vi "CleanUp.vi"(8 "error in (no error)":errorcluster, 11 "Prueba08 in":refnum<class "Prueba031.lvclass">) -> (0 "error out":errorcluster, 3 "Prueba08 out":refnum<class "Prueba031.lvclass">)   [LabVIEW 2019, in "Prueba031.lvclass"]
uses:
  Prueba031.lvclass
  Prueba031.lvclass/Prueba031.ctl
panel:
  out "Tabla_int":string[][](array[string])
  out "Tabla_ext":string[][](array[string])
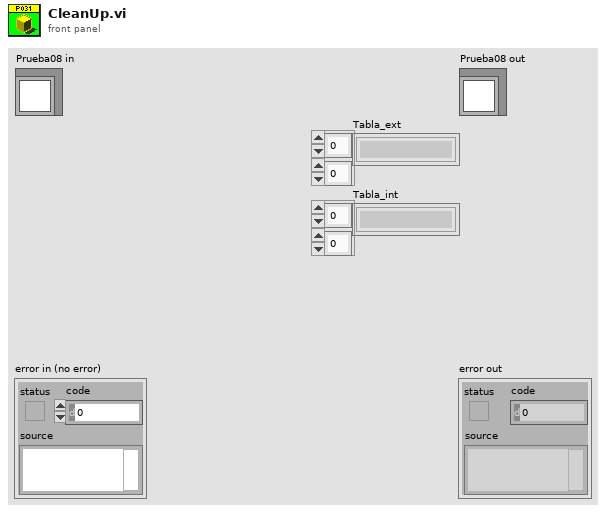
[diagram p1: front panel]
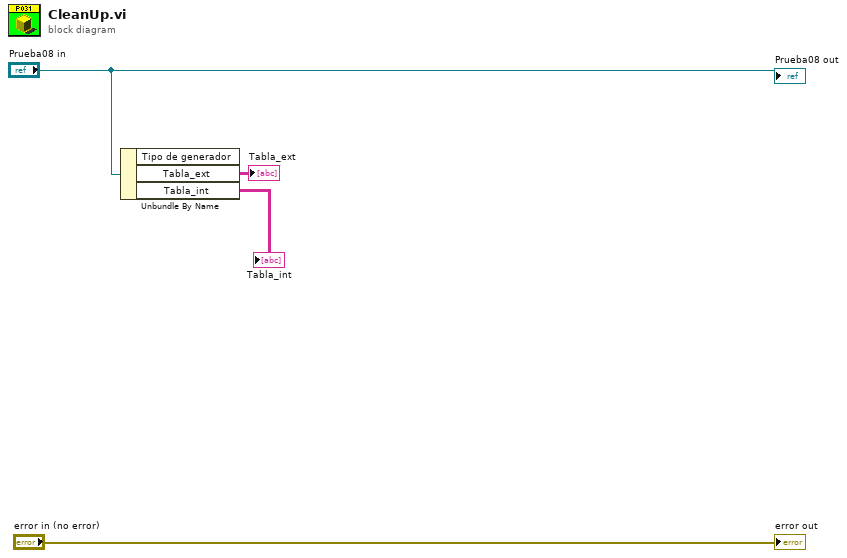
[diagram p0: block diagram]
diagram:
  n1 = Unbundle By Name("Prueba08 in") -> ("Tabla_ext"=→"Tabla_ext":string[][], "Tabla_int"=→"Tabla_int":string[][])  [unwired: 1 out]
  "error out" <- "error in (no error)"
  "Prueba08 out" <- "Prueba08 in"
